vi "Max Bin Read.vi"(0 "FPGA VI Reference In":refnum<k20>, 3 "error in":errorcluster) -> (14 "Max Bin":i32, 15 "Max Amp":fxp<+,46,22>, 16 "Prev Bin":i32, 17 "Prev Amp":fxp<+,46,22> format="%.41g", 18 "Next Bin":i32, 19 "Next Amp":fxp<+,46,22> format="%.41g")   [LabVIEW 2014]
uses:
  <vilib>/Utility/error.llb/Error Cluster From Error Code.vi
  <vilib>/rvi/errors/niLvFpgaAdjustHostInterfaceError.vi
  <vilib>/rvi/interface/nirviMethod/nirviMethod.xnode
  <vilib>/FPGAPlugInAG/Dynamic/niLvFpga_ReadFifo_Dynamic.vi
  <vilib>/rvi/errors/niLvFpgaMergeErrorWithErrorCode.vi
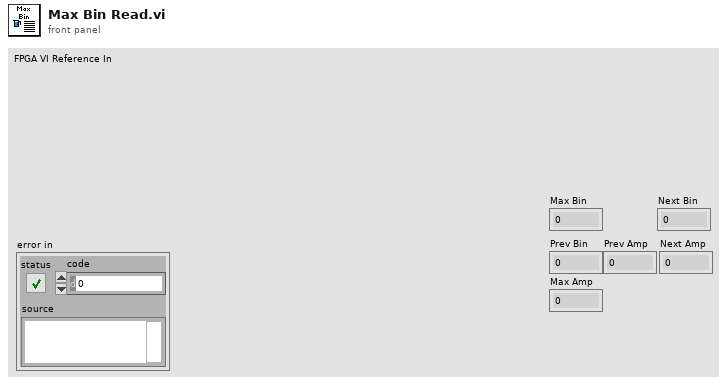
[diagram p1: front panel]
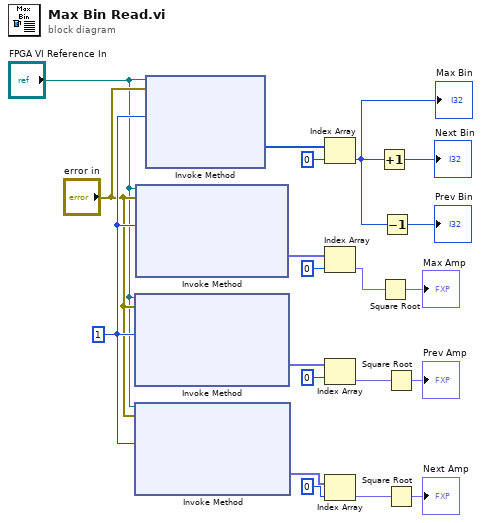
[diagram p0: block diagram]
diagram:
  w20 = u32 1 ("Number of Elements")
  n1 = xnode "Invoke Method"("FPGA VI Reference In"="FPGA VI Reference In", "error in"="error in", "Number of Elements"=w20) -> ("Data"=w14:fxp<+,44,44>[])  [unwired: 1 in, 3 out]
  n2 = xnode "Invoke Method"("FPGA VI Reference In"="FPGA VI Reference In", "error in"="error in", "Number of Elements"=w20) -> ("Data"=w12:fxp<+,44,44>[])  [unwired: 1 in, 3 out]
  n3 = xnode "Invoke Method"("FPGA VI Reference In"="FPGA VI Reference In", "error in"="error in", "Number of Elements"=w20) -> ("Data"=w16:fxp<+,44,44>[])  [unwired: 1 in, 3 out]
  n4 = xnode "Invoke Method"("FPGA VI Reference In"="FPGA VI Reference In", "error in"="error in", "Number of Elements"=w20) -> ("Data"=w19:i32[])  [unwired: 1 in, 3 out]
  n5 = Index Array(array=w19, index=0) -> (element=w8:i32)
  "Max Bin" <- w8
  n6 = Index Array(array=w16, index=0) -> (element=w7:fxp<+,44,44>)
  n7 = Index Array(array=w14, index=0) -> (element=w5:fxp<+,44,44>)
  n8 = Index Array(array=w12, index=0) -> (element=w3:fxp<+,44,44>)
  n9 = Increment(x=w8) -> (x+1=→"Next Bin":i32)
  n10 = Square Root(x=w7) -> (sqrt(x)=→"Max Amp":fxp<+,46,22>)
  n11 = Decrement(x=w8) -> (x-1=→"Prev Bin":i32)
  n12 = Square Root(x=w5) -> (sqrt(x)=→"Prev Amp":fxp<+,46,22>)
  n13 = Square Root(x=w3) -> (sqrt(x)=→"Next Amp":fxp<+,46,22>)
